vi "GetAxisInfo.vi"(0 "axis in":cluster{"keyHandle":u32, "nodeId":u16}={"keyHandle"=0, "nodeId"=1}, 11 "error in (no error)":errorcluster) -> (4 "axis out":cluster{"keyHandle":u32, "nodeId":u16}={"keyHandle"=0, "nodeId"=1}, 6 "axis state":T2(ring), 8 "targetReached":i32, 10 "axis data":T1, 15 "error out":errorcluster)   [LabVIEW 2018]
doc: "<B>GetAxisInfos</B> reads the actual position, velocity and current from the device and looks if the target is reached."
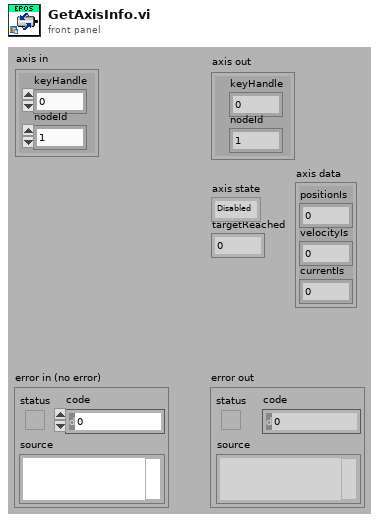
[diagram p1: front panel]
types:
  T1 = cluster{"positionIs":i32, "velocityIs":i32, "currentIs":i16}
  T2 = enum16{"Disabled", "Enabled", "Quickstop", "Fault"}
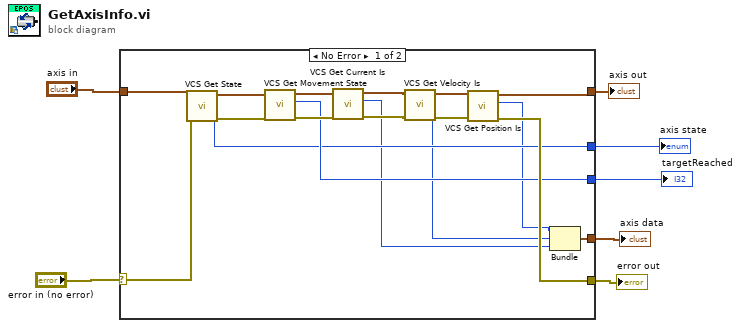
[diagram p0: block diagram]
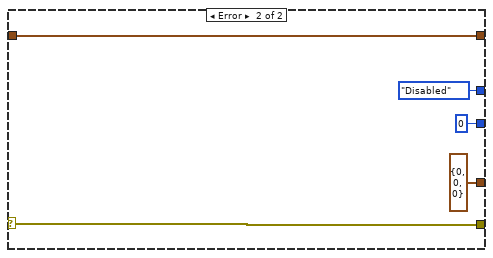
[diagram p2: hidden frame]
diagram:
  n1 = case shown="No Error" "error in (no error)" {
    selector: "error in (no error)" -> [w15 w30]
    tunnel: [w21 w30] -> w6
    tunnel: [w22 w29] -> w5
    tunnel: "axis in" -> [w16 w29]
    tunnel: [w17 0 ("targetReached")] -> w3
    tunnel: [w12 T2."Disabled" ("state")] -> w2
    tunnel: [w8 T1 {"positionIs"=0, "velocityIs"=0, "currentIs"=0}] -> w1
    frame No Error {
      n2 = call "VCS Get State.vi"("error in (no error)"=w15, "axis in"=w16) -> ("error out"=w13:errorcluster, "state"=w12:T2, "axis out"=w14:cluster{"keyHandle":u32, "nodeId":u16})  [unwired: 7 in]
      n3 = call "VCS Get Movement State.vi"("error in (no error)"=w13, "axis in"=w14) -> ("error out"=w18:errorcluster, "targetReached"=w17:i32, "axis out"=w25:cluster{"keyHandle":u32, "nodeId":u16})  [unwired: 7 in]
      n4 = call "VCS Get Current Is.vi"("error in (no error)"=w18, "axis in"=w25) -> ("error out"=w19:errorcluster, "currentIs"=w9:i16, "axis out"=w24:cluster{"keyHandle":u32, "nodeId":u16})  [unwired: 7 in]
      n5 = call "VCS Get Velocity Is.vi"("error in (no error)"=w19, "axis in"=w24) -> ("error out"=w20:errorcluster, "velocityIs"=w10:i32, "axis out"=w23:cluster{"keyHandle":u32, "nodeId":u16})  [unwired: 7 in]
      n6 = call "VCS Get Position Is.vi"("error in (no error)"=w20, "axis in"=w23) -> ("error out"=w21:errorcluster, "positionIs"=w11:i32, "axis out"=w22:cluster{"keyHandle":u32, "nodeId":u16})  [unwired: 7 in]
      n7 = Bundle("positionIs"=w11, "velocityIs"=w10, "currentIs"=w9) -> (w8:T1)  [unwired: 1 in]
    }
    frame Error {
    }
  }
  "error out" <- w6
  "axis out" <- w5
  "targetReached" <- w3
  "axis state" <- w2
  "axis data" <- w1
